vi "Read Laser Enable.vi"(8 "error in (no error)":errorcluster, 11 "Set f0 MSG in":refnum<class "Set Las Enable MSG.lvclass">) -> (0 "error out":errorcluster, 2 "Laser Enable":bool[](array[boolean]), 3 "Set f0 MSG out":refnum<class "Set Las Enable MSG.lvclass">)   [LabVIEW 2014, in "ePAS Library.lvlib" / "Set Las Enable MSG.lvclass"]
uses:
  Set Las Enable MSG.lvclass
  Set Las Enable MSG.lvclass/Set Las Enable MSG.ctl
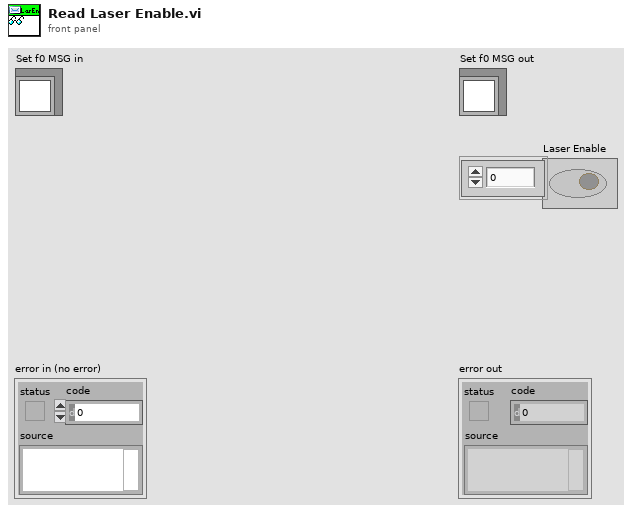
[diagram p1: front panel]
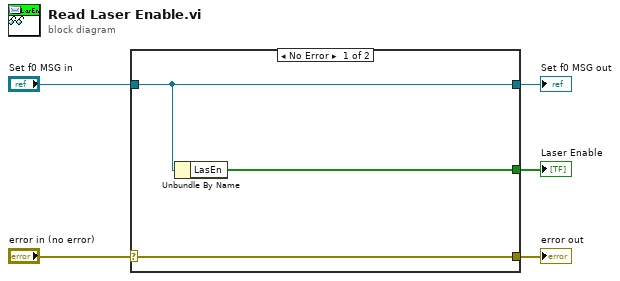
[diagram p0: block diagram]
diagram:
  n1 = case shown="No Error" "error in (no error)" {
    selector: "error in (no error)" -> [w8 w9]
    tunnel: [w8 w9] -> w4
    tunnel: [w7 w10] -> w2
    tunnel: "Set f0 MSG in" -> [w7 w10]
    tunnel: [w6 _] -> w1
    frame No Error {
      n2 = Unbundle By Name(w7) -> ("LasEn"=w6:bool[])
    }
    frame Error {
    }
  }
  "error out" <- w4
  "Set f0 MSG out" <- w2
  "Laser Enable" <- w1
